vi "Destroy Message Transport.vi"(8 "error in":errorcluster, 11 "UserEventMessageTransport":refnum<class "UserEventMessageTransport.lvclass">) -> (0 "error out":errorcluster, 3 "UserEventMessageTransport":refnum<class "UserEventMessageTransport.lvclass">)   [LabVIEW 2016, in "UserEventMessageTransport.lvclass"]
uses:
  UserEventMessageTransport.lvclass
panel:
  # "INPUTS"
  # "OUTPUTS"
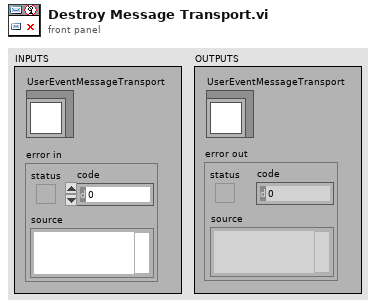
[diagram p1: front panel]
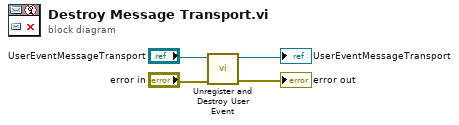
[diagram p0: block diagram]
diagram:
  n1 = call "Unregister and Destroy User Event.vi"("error in"="error in", "UserEventMessageTransport"="UserEventMessageTransport") -> ("error out"=→"error out":errorcluster, "UserEventMessageTransport"=→"UserEventMessageTransport":refnum<class "UserEventMessageTransport.lvclass">)  [unwired: 8 in]
